vi "拟合切线显示.vi"(3 "计算参数 in":T1) -> (0 "计算参数 out":T1, 2 "Array out":dbl[](array[numeric]))   [LabVIEW 2013]
doc: "这个函数生成ts1到ts2之间的纵坐标的值数组，不改变计算参数的值"
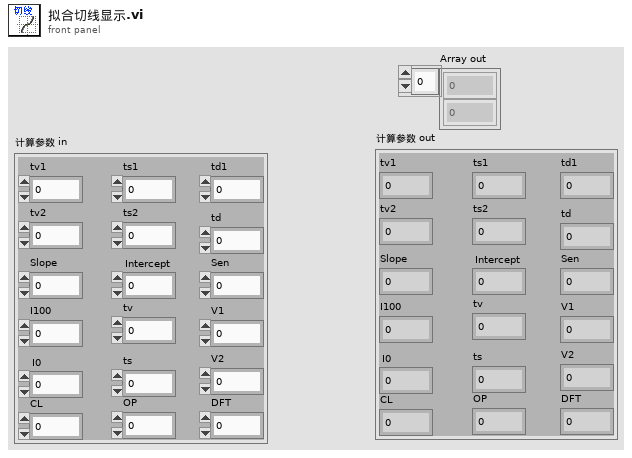
[diagram p1: front panel]
types:
  T1 = cluster{"tv1":dbl, "tv2":dbl, "tv":dbl, "ts1":dbl, "ts2":dbl, "ts":dbl, "td1":dbl, "td":dbl, "Slope":dbl, "Intercept":dbl, "I100":dbl, "I0":dbl, "Sen":dbl, "V1":dbl, "V2":dbl, "CL":dbl, "OP":dbl, "DFT":dbl}
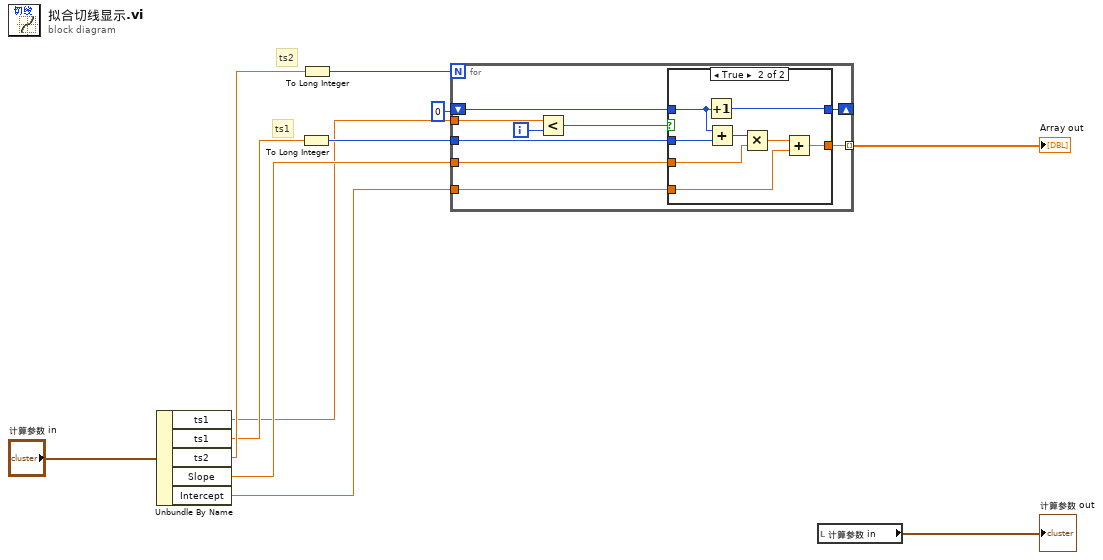
[diagram p0: block diagram]
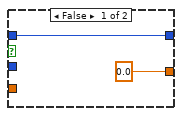
[diagram p2: hidden frame]
diagram:
  # "ts1"
  # "ts2"
  n1 = Unbundle By Name("计算参数 in") -> ("ts1"=w2:dbl, "ts1"=w6:dbl, "ts2"=w10:dbl, "Slope"=w5:dbl, "Intercept"=w7:dbl)
  n2 = To Long Integer(number=w6) -> (32bit integer=w4:i32)
  n3 = To Long Integer(number=w10) -> (32bit integer=w8:i32)
  n4 = for {
    N: w8 -> [_]
    tunnel: w5 -> [w19]
    tunnel: w7 -> [w18]
    tunnel: [w17] -> w9 mode=indexing
    tunnel: w4 -> [w16]
    shift-right: [w14] -> _
    shift-left: 0 -> [w13]
    tunnel: w2 -> [w12]
    i -> [w15]
    n5 = Less?(x=w12, y=w15) -> (x < y?=w20:bool)
    n6 = case shown="True" w20 {
      tunnel: w19 -> [_ w28]
      tunnel: w16 -> [_ w27]
      tunnel: w18 -> [_ w26]
      tunnel: [0.0 w25] -> w17
      tunnel: [w22 w24] -> w14
      tunnel: w13 -> [w22 w23]
      frame False {
      }
      frame True {
        n7 = Increment(x=w23) -> (x+1=w24:i32)
        n8 = Add(x=w23, y=w27) -> (x+y=w30:i32)
        n9 = Multiply(x=w30, y=w28) -> (x*y=w29:dbl)
        n10 = Add(x=w29, y=w26) -> (x+y=w25:dbl)
      }
    }
  }
  "Array out" <- w9
  n11 = local read "计算参数 in"() -> (→"计算参数 out":T1)
